vi "execute.vi"(8 "error in (no error)":errorcluster, 9 "image assembler in":refnum<class "GenericComponent.lvclass">, 10 "imaging mode in":refnum<class "GenericComponent.lvclass">, 11 "adapter in":refnum<class "AdapterDL091215ImagingModeToImageAssembler.lvclass">) -> (0 "error out":errorcluster, 1 "image assembler out":refnum<class "GenericComponent.lvclass">, 2 "imaging mode out":refnum<class "GenericComponent.lvclass">, 3 "adapter out":refnum<class "AdapterDL091215ImagingModeToImageAssembler.lvclass">)   [LabVIEW 2010, in "AdapterDL091215ImagingModeToImageAssembler.lvclass"]
uses:
  AdapterDL091215ImagingModeToImageAssembler.lvclass
  common/classes/GenericComponent/GenericComponent/GenericComponent.lvclass
  ImageAssembler/ImageAssemblerMG090623Binning/ImageAssemblerMG090623Binning/ImageAssemblerMG090623Binning.lvclass
  ImagingMode/ImagingModeMG091111IntrinsicImaging/ImagingModeMG091111IntrinsicImaging/ImagingModeMG091111IntrinsicImaging.lvclass
panel:
  # "imaging mode: ImagingModeMG091111IntrinsicImaging\nimage assembler: ImageAssemblerMG090623Binning"
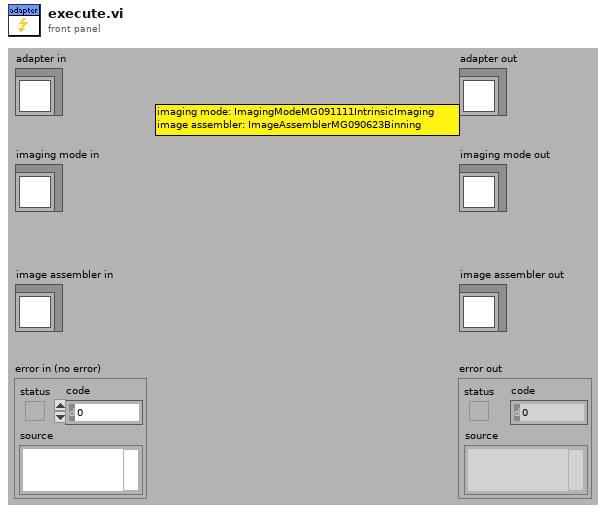
[diagram p1: front panel]
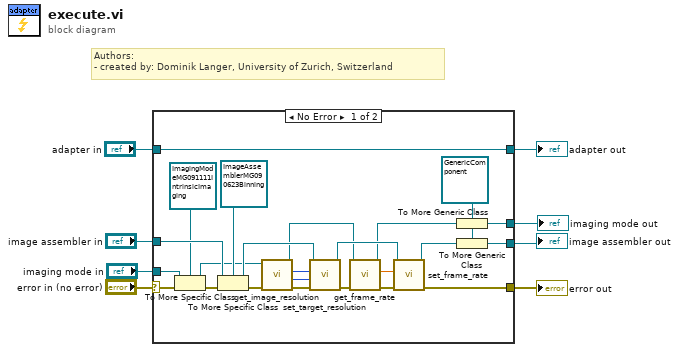
[diagram p0: block diagram]
diagram:
  # "Authors: \n- created by: Dominik Langer, University of Zurich, Switzerland"
  n1 = case shown="No Error" "error in (no error)" {
    selector: "error in (no error)" -> [w32 w33]
    tunnel: "imaging mode in" -> [w18 w34]
    tunnel: "image assembler in" -> [w30 w35]
    tunnel: "adapter in" -> [w29 w36]
    tunnel: [w29 w36] -> w4
    tunnel: [w28 w35] -> w3
    tunnel: [w26 w34] -> w2
    tunnel: [w14 w33] -> w1
    frame No Error {
      w27 = refnum<class "GenericComponent.lvclass"> refnum ("GenericComponent.lvclass")
      n2 = To More Specific Class(target class=refnum<class "ImagingModeMG091111IntrinsicImaging.lvclass"> refnum ("ImagingModeMG091111IntrinsicImaging.lvclass"), reference=w18, error in=w32) -> (specific class reference=w17:refnum<class "ImagingModeMG091111IntrinsicImaging.lvclass">, error out=w31:errorcluster)
      n3 = To More Specific Class(target class=refnum<class "ImageAssemblerMG090623Binning.lvclass"> refnum ("ImageAssemblerMG090623Binning.lvclass"), reference=w30, error in=w31) -> (specific class reference=w23:refnum<class "ImageAssemblerMG090623Binning.lvclass">, error out=w22:errorcluster)
      n4 = call-dynamic "get_image_resolution.vi"("error in (no error)"=w22, "ScanModeMG091111IntrinsicImaging in"=w17) -> ("error out"=w21:errorcluster, "ImageHeight"=w20:i32, "ImageWidth"=w19:i32, "ScanModeMG091111IntrinsicImaging out"=w11:refnum<class "ImagingModeMG091111IntrinsicImaging.lvclass">)  [unwired: 6 in]
      n5 = call-dynamic "set_target_resolution.vi"("error in (no error)"=w21, "y"=w20, "x"=w19, "MG090623BinningImageAssembler.lvclass in"=w23) -> ("error out"=w13:errorcluster, "MG090623BinningImageAssembler.lvclass out"=w16:refnum<class "ImageAssemblerMG090623Binning.lvclass">)  [unwired: 6 in]
      n6 = call-dynamic "get_frame_rate.vi"("error in (no error)"=w13, "ScanModeMG091111IntrinsicImaging in"=w11) -> ("error out"=w12:errorcluster, "frame rate"=w9:dbl[unit], "ScanModeMG091111IntrinsicImaging out"=w10:refnum<class "ImagingModeMG091111IntrinsicImaging.lvclass">)  [unwired: 7 in]
      n7 = call-dynamic "set_frame_rate.vi"("error in (no error)"=w12, "frame rate"=w9, "MG090623BinningImageAssembler.lvclass in"=w16) -> ("error out"=w14:errorcluster, "MG090623BinningImageAssembler.lvclass out"=w15:refnum<class "ImageAssemblerMG090623Binning.lvclass">)  [unwired: 7 in]
      n8 = To More Generic Class(target class=w27, reference=w10) -> (generic class reference=w26:refnum<class "GenericComponent.lvclass">)
      n9 = To More Generic Class(target class=w27, reference=w15) -> (generic class reference=w28:refnum<class "GenericComponent.lvclass">)
    }
    frame Error {
    }
  }
  "error out" <- w1
  "adapter out" <- w4
  "imaging mode out" <- w2
  "image assembler out" <- w3
